vi "close connection.vi"(8 "error in (no error)":errorcluster, 11 "EMTestCWS500N in":refnum<class "EMTestCWS500N.lvclass">) -> (0 "error out":errorcluster, 3 "EMTestCWS500N out":refnum<class "EMTestCWS500N.lvclass">)   [LabVIEW 2013, in "EMTestCWS500N.lvclass"]
uses:
  EMTestCWS500N.lvclass
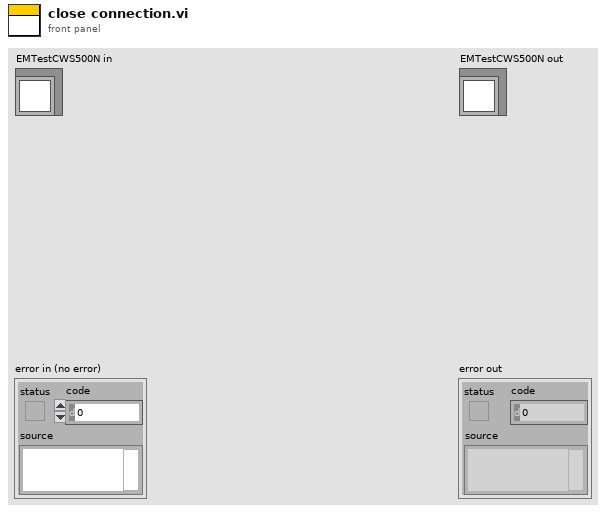
[diagram p1: front panel]
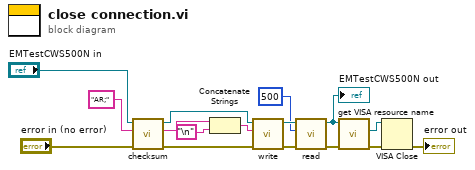
[diagram p0: block diagram]
diagram:
  n1 = call-dynamic "checksum.vi"("error in (no error)"="error in (no error)", "input"="AR;", "EMTestCWS500N in"="EMTestCWS500N in") -> ("error out"=w12:errorcluster, "output"=w2:string, "EMTestCWS500N out"=w13:refnum<class "EMTestCWS500N.lvclass">)  [unwired: 6 in]
  n2 = Concatenate Strings(w2, "\n") -> (w1:string)
  n3 = call-dynamic "write.vi"("error in (no error)"=w12, "String to send"=w1, "EMTestCWS500N in"=w13) -> ("error out"=w7:errorcluster, "EMTestCWS500N out"=w8:refnum<class "EMTestCWS500N.lvclass">)  [unwired: 7 in]
  n4 = call-dynamic "read.vi"("error in (no error)"=w7, "timeout (ms)"=500, "EMTestCWS500N in"=w8) -> ("error out"=w5:errorcluster, "EMTestCWS500N out"=w4:refnum<class "EMTestCWS500N.lvclass">)  [unwired: 6 in, 1 out]
  "EMTestCWS500N out" <- w4
  n5 = call-dynamic "get VISA resource name.vi"("error in (no error)"=w5, "DeviceInterface (Eingang)"=w4) -> ("error out"=w9:errorcluster, "VISA resource name"=w10:refnum<visa-resource-name>)  [unwired: 7 in, 1 out]
  n6 = VISA Close(VISA resource name=w10, error in (no error)=w9) -> (error out=→"error out":errorcluster)
